vi "GetSubscriptionDeviceInfo.vi"() -> ()   [LabVIEW 2013]
uses:
  Shared/MySQL/Preset Query Enum.ctl
panel:
  out "Data read by TCP":string[](array[string])
  out "TCP Ports":refnum<k5>[](array[refnum])
  in  "error in (no error)":errorcluster
  out "error out":errorcluster
  in  "Devices and Variables":string[][](array[string])=[["device", "variablename", "defaultvalue", "startvalue", "endvalue"], ["TREX Mode Imager", "Exposure", "0.1", "0.1", "0.1"], ["TREX Mode Imager", "Gain", "0.1", "0.1", "0.1"], ["Cam1", "Exposure", "0.1", "0.1", "0.1"]]
  out "data":string[][](array[string])
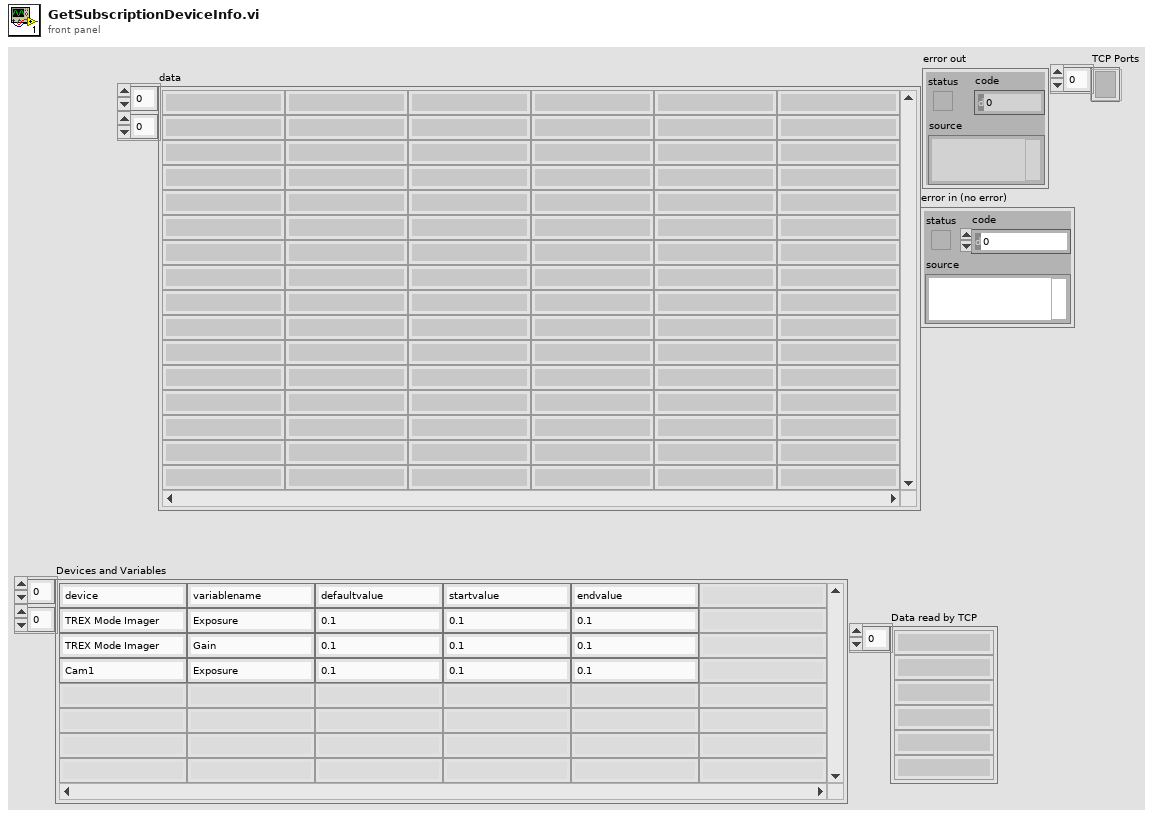
[diagram p1: front panel]
types:
  T1 = typedef "Preset Query Enum.ctl" = enum16{"Get Locations", "Get all IPs and MACs", "Get classes", "Get expt variables to set at scanstart for particular device", "Get expt devices and variables with start values", "Get expt devices and variables (with data to get)", "Get expt devices with data to get", "Get Expt devices and GUIs", "Get all devices basic properties", "Get Virtual Devices Core Info", "Get Expt names", "Get experiment basic properties", "Get experiment alarm variables", "Get MC Ports", "Get device network comm port", "Get devicetype lvclass path", "Get basic device properties", "Get Init Order", "Get all setable variables of a device", "Get device variable aliases", "Get force values of all settable variables", "Get all variables of a devicetype", "Get all variables of a device", "Get plotter details", "Get Saved Scans", "Get Scan Info", "GetGeneralGUIs", "Get expt for plotter", "Get plotter IDs from expt", "Get all devices", "Get all Virtual Devices", "Get all aliases", "Get variable and device info for Virtual Device", "GetItemLocatorIP", "Get IPs for GUIs", "Get DeviceType from Device", "GetLocalPortRange", "GetDevicePresetVariables", "Get Device Configuration", "GetAllPresetNames", "GetAllConfigurationNames", "GetPresetDeviceNames"}
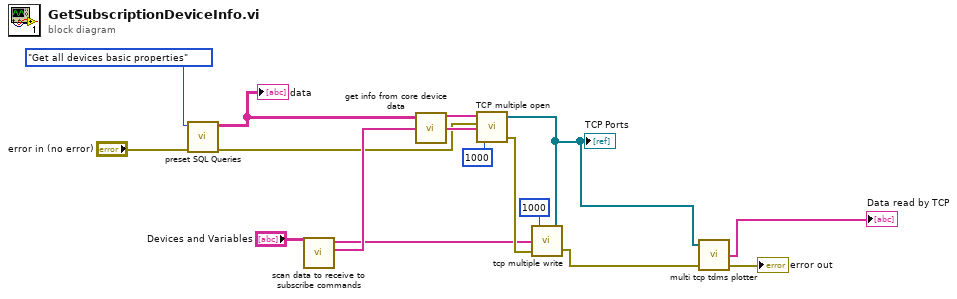
[diagram p0: block diagram]
diagram:
  n1 = call "preset SQL Queries.vi"("error in (no error)"="error in (no error)", "Preset Query"=Preset_Query_Enum."Get all devices basic properties") -> ("error out"=w5:errorcluster, "data"=w15:string[][])  [unwired: 7 in, 1 out]
  "data" <- w15
  n2 = call "scan data to receive to subscribe commands.vi"("ScanData to receive"="Devices and Variables") -> ("devices"=w10:string[], "Subscribe commands"=w7:string[])  [unwired: 8 in, 1 out]
  n3 = call "get info from core device data.vi"("devices to get data from"=w10, "All Devices Core Info"=w15) -> ("Ports"=w13:string[], "IP Addresses"=w14:string[])  [unwired: 2 in]
  n4 = call "TCP multiple open.vi"("timeout ms (60000)"=1000, "Ports"=w13, "error in 1 (no error)"=w5, "IP Addresses"=w14) -> ("error out"=w8:errorcluster, "Array"=w4:refnum<k5>[])  [unwired: 1 out]
  "TCP Ports" <- w4
  n5 = call "tcp multiple write.vi"("Connection ID array"=w4, "error in 1 (no error)"=w8, "messages to send"=w7, "timeout ms (25000)"=1000) -> ("error out"=w3:errorcluster)
  n6 = call "multi tcp tdms plotter.vi"("error in"=w3, "TCP connections"=w4) -> ("error out"=→"error out":errorcluster, "replies"=→"Data read by TCP":string[])  [unwired: 2 in]
